vi "SkipVISANumbOfBytesWarning.vi"(8 "error in (no error)":errorcluster, 11 "VISA resource name":refnum<visa-resource-name>) -> (0 "error out":errorcluster, 3 "dup VISA resource name":refnum<visa-resource-name>)   [LabVIEW 2021]
doc: "Dieses VI löscht die VISA Warning mit der Nummer = 1073676294 aus dem ErrorCluster.\n(The number of bytes transferred is equal to the input count)\nInteressiert eigentlich niemanden und ist lästig.\n\nZühlke Engineering AG\n30.Juni 2003"
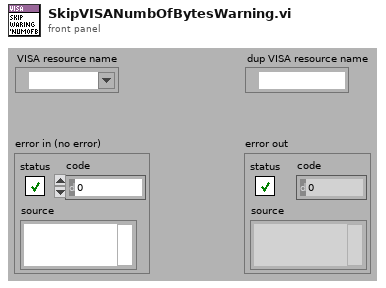
[diagram p1: front panel]
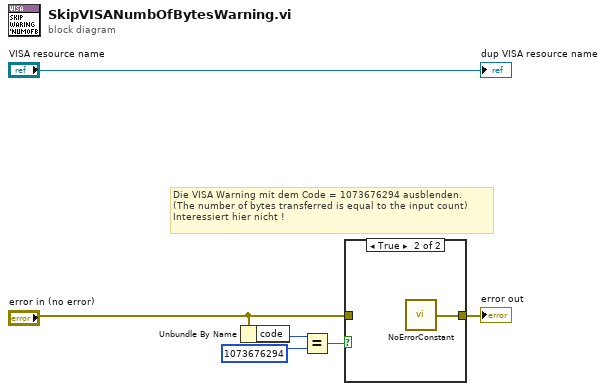
[diagram p0: block diagram]
diagram:
  # "Die VISA Warning mit dem Code = 1073676294 ausblenden.\n(The number of bytes transferred is equal to the input count)\nInteressiert hier nicht !"
  n1 = Unbundle By Name("error in (no error)") -> ("code"=w6:i32)
  n2 = Equal?(x=w6, y=1073676294) -> (x = y?=w4:bool)
  n3 = case shown="True" w4 {
    tunnel: "error in (no error)" -> [w7 _]
    tunnel: [w7 w8] -> w2
    frame False {
    }
    frame True {
      n4 = call "NoErrorConstant.vi"() -> ("error out (no Error)"=w8:errorcluster)  [unwired: 5 in]
    }
  }
  "error out" <- w2
  "dup VISA resource name" <- "VISA resource name"
